vi "Sort 2D-Array.vi"(1 "Sort Order (0->9)":enum16{"0 --> 9", "9 --> 0"}(ring), 2 "Search Parameters":T1, 7 "2D-String-Array_in":string[][](array[string])=[["45245,25", "Hallo", "Eier"], ["45245,36", "Ballo", "Mehl"], ["45245,84", "Lallo", "Zucker"], ["245", "Trallo", "Salz"], ["45", "Knallo", "Bier"]]) -> (8 "2D-String-Array_SortedByColumn":string[][](array[string]))   [LabVIEW 2022 SP3, in "hse-misc.lvlib"]
doc: "Sorts a 2D string array by the column declared in <b>Search parameters</b> and by <b>Sort Order</b>.\n\n\n\n____\nHAMPEL SOFTWARE ENGINEERING v3.8.0 (2023-12-18 14:41)"
uses:
  hse-misc.lvlib
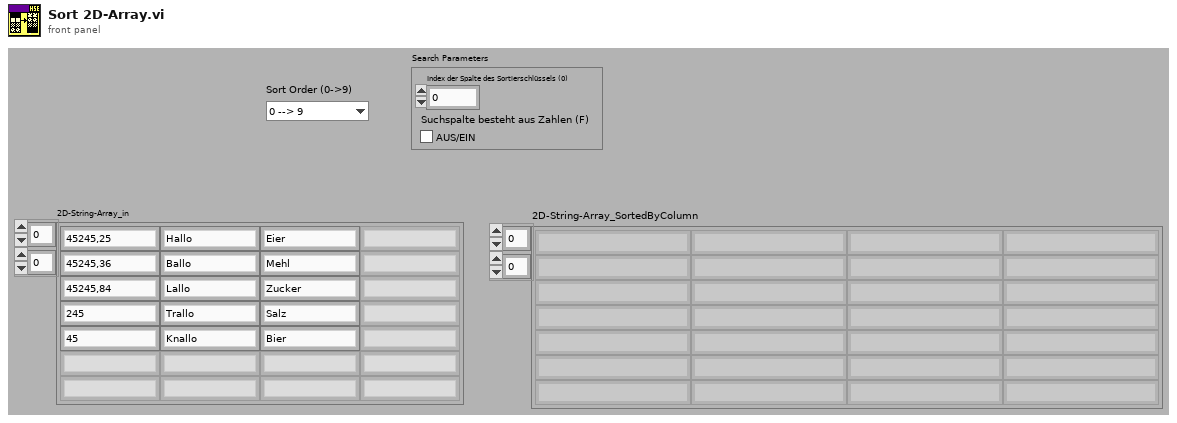
[diagram p1: front panel]
types:
  T1 = cluster{"Index der Spalte des Sortierschlüssels (0)":i32, "Suchspalte besteht aus Zahlen (F)":bool}
  T2 = cluster{"[0]":string, "[1]":string, "[2]":string, "[3]":string, "[4]":string, "[5]":string, "[6]":string, "[7]":string, "[8]":string, "[9]":string, "[10]":string, "[11]":string, "[12]":string, "[13]":string, "[14]":string, "[15]":string, "[16]":string, "[17]":string, "[18]":string, "[19]":string, "[20]":string, "[21]":string, "[22]":string, "[23]":string, "[24]":string, "[25]":string, "[26]":string, "[27]":string, "[28]":string, "[29]":string, "[30]":string, "[31]":string, "[32]":string, "[33]":string, "[34]":string, "[35]":string, "[36]":string, "[37]":string, "[38]":string, "[39]":string, "[40]":string, "[41]":string, "[42]":string, "[43]":string, "[44]":string, "[45]":string, "[46]":string, "[47]":string, "[48]":string, "[49]":string, "[50]":string, "[51]":string, "[52]":string, "[53]":string, "[54]":string, "[55]":string, "[56]":string, "[57]":string, "[58]":string, "[59]":string, "[60]":string, "[61]":string, "[62]":string, "[63]":string, "[64]":string, "[65]":string, "[66]":string, "[67]":string, "[68]":string, "[69]":string, "[70]":string, "[71]":string, "[72]":string, "[73]":string, "[74]":string, "[75]":string, "[76]":string, "[77]":string, "[78]":string, "[79]":string, "[80]":string, "[81]":string, "[82]":string, "[83]":string, "[84]":string, "[85]":string, "[86]":string, "[87]":string, "[88]":string, "[89]":string, "[90]":string, "[91]":string, "[92]":string, "[93]":string, "[94]":string, "[95]":string, "[96]":string, "[97]":string, "[98]":string, "[99]":string}
  T3 = cluster{dbl, cluster{"[0]":string, "[1]":string, "[2]":string, "[3]":string, "[4]":string, "[5]":string, "[6]":string, "[7]":string, "[8]":string, "[9]":string, "[10]":string, "[11]":string, "[12]":string, "[13]":string, "[14]":string, "[15]":string, "[16]":string, "[17]":string, "[18]":string, "[19]":string, "[20]":string, "[21]":string, "[22]":string, "[23]":string, "[24]":string, "[25]":string, "[26]":string, "[27]":string, "[28]":string, "[29]":string, "[30]":string, "[31]":string, "[32]":string, "[33]":string, "[34]":string, "[35]":string, "[36]":string, "[37]":string, "[38]":string, "[39]":string, "[40]":string, "[41]":string, "[42]":string, "[43]":string, "[44]":string, "[45]":string, "[46]":string, "[47]":string, "[48]":string, "[49]":string, "[50]":string, "[51]":string, "[52]":string, "[53]":string, "[54]":string, "[55]":string, "[56]":string, "[57]":string, "[58]":string, "[59]":string, "[60]":string, "[61]":string, "[62]":string, "[63]":string, "[64]":string, "[65]":string, "[66]":string, "[67]":string, "[68]":string, "[69]":string, "[70]":string, "[71]":string, "[72]":string, "[73]":string, "[74]":string, "[75]":string, "[76]":string, "[77]":string, "[78]":string, "[79]":string, "[80]":string, "[81]":string, "[82]":string, "[83]":string, "[84]":string, "[85]":string, "[86]":string, "[87]":string, "[88]":string, "[89]":string, "[90]":string, "[91]":string, "[92]":string, "[93]":string, "[94]":string, "[95]":string, "[96]":string, "[97]":string, "[98]":string, "[99]":string}}
  T4 = cluster{dbl, cluster{"[0]":string, "[1]":string, "[2]":string, "[3]":string, "[4]":string, "[5]":string, "[6]":string, "[7]":string, "[8]":string, "[9]":string, "[10]":string, "[11]":string, "[12]":string, "[13]":string, "[14]":string, "[15]":string, "[16]":string, "[17]":string, "[18]":string, "[19]":string, "[20]":string, "[21]":string, "[22]":string, "[23]":string, "[24]":string, "[25]":string, "[26]":string, "[27]":string, "[28]":string, "[29]":string, "[30]":string, "[31]":string, "[32]":string, "[33]":string, "[34]":string, "[35]":string, "[36]":string, "[37]":string, "[38]":string, "[39]":string, "[40]":string, "[41]":string, "[42]":string, "[43]":string, "[44]":string, "[45]":string, "[46]":string, "[47]":string, "[48]":string, "[49]":string, "[50]":string, "[51]":string, "[52]":string, "[53]":string, "[54]":string, "[55]":string, "[56]":string, "[57]":string, "[58]":string, "[59]":string, "[60]":string, "[61]":string, "[62]":string, "[63]":string, "[64]":string, "[65]":string, "[66]":string, "[67]":string, "[68]":string, "[69]":string, "[70]":string, "[71]":string, "[72]":string, "[73]":string, "[74]":string, "[75]":string, "[76]":string, "[77]":string, "[78]":string, "[79]":string, "[80]":string, "[81]":string, "[82]":string, "[83]":string, "[84]":string, "[85]":string, "[86]":string, "[87]":string, "[88]":string, "[89]":string, "[90]":string, "[91]":string, "[92]":string, "[93]":string, "[94]":string, "[95]":string, "[96]":string, "[97]":string, "[98]":string, "[99]":string}}[]
  T5 = cluster{"[0]":string, "[1]":string, "[2]":string, "[3]":string, "[4]":string, "[5]":string, "[6]":string, "[7]":string, "[8]":string, "[9]":string, "[10]":string, "[11]":string, "[12]":string, "[13]":string, "[14]":string, "[15]":string, "[16]":string, "[17]":string, "[18]":string, "[19]":string, "[20]":string, "[21]":string, "[22]":string, "[23]":string, "[24]":string, "[25]":string, "[26]":string, "[27]":string, "[28]":string, "[29]":string, "[30]":string, "[31]":string, "[32]":string, "[33]":string, "[34]":string, "[35]":string, "[36]":string, "[37]":string, "[38]":string, "[39]":string, "[40]":string, "[41]":string, "[42]":string, "[43]":string, "[44]":string, "[45]":string, "[46]":string, "[47]":string, "[48]":string, "[49]":string, "[50]":string, "[51]":string, "[52]":string, "[53]":string, "[54]":string, "[55]":string, "[56]":string, "[57]":string, "[58]":string, "[59]":string, "[60]":string, "[61]":string, "[62]":string, "[63]":string, "[64]":string, "[65]":string, "[66]":string, "[67]":string, "[68]":string, "[69]":string, "[70]":string, "[71]":string, "[72]":string, "[73]":string, "[74]":string, "[75]":string, "[76]":string, "[77]":string, "[78]":string, "[79]":string, "[80]":string, "[81]":string, "[82]":string, "[83]":string, "[84]":string, "[85]":string, "[86]":string, "[87]":string, "[88]":string, "[89]":string, "[90]":string, "[91]":string, "[92]":string, "[93]":string, "[94]":string, "[95]":string, "[96]":string, "[97]":string, "[98]":string, "[99]":string}[]
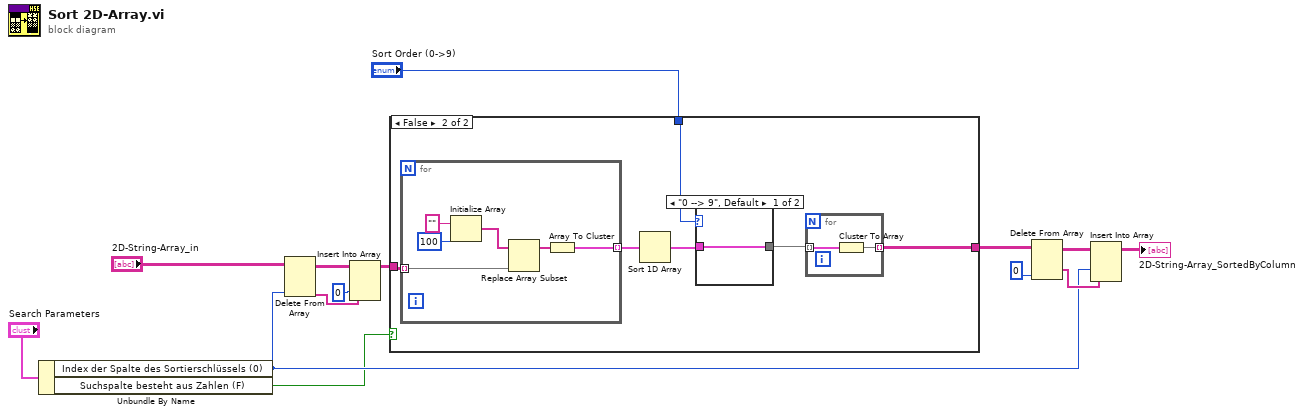
[diagram p0: block diagram]
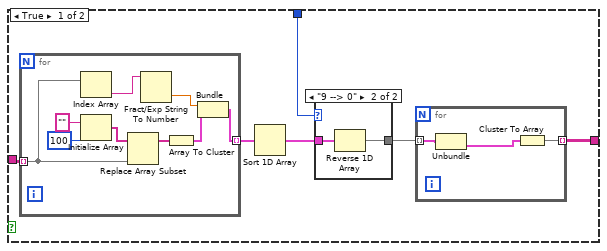
[diagram p2: hidden frame]
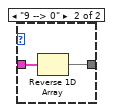
[diagram p4: hidden frame]
diagram:
  n1 = Unbundle By Name("Search Parameters") -> ("Index der Spalte des Sortierschlüssels (0)"=w4:i32, "Suchspalte besteht aus Zahlen (F)"=w3:bool)
  n2 = Delete From Array(array="2D-String-Array_in", index (col)=w4) -> (deleted portion=w6:string[], array with subset deleted=w14:string[][])  [unwired: 2 in]
  n3 = Insert Into Array(array=w14, index (col)=0 ("Deaktivierter Index (Spalte)"), new element=w6) -> (w12:string[][])  [unwired: 1 in]
  n4 = case shown="False" w3 {
    tunnel: w12 -> [w18 w40]
    tunnel: [w17 w39] -> w8
    tunnel: "Sort Order (0->9)" -> [w15 w36]
    frame True {
      n5 = for {
        tunnel: w18 -> [w28] mode=indexing
        tunnel: [w25] -> w20 mode=indexing
        n6 = Index Array(array=w28) -> (element=w27:string)  [unwired: 1 in]
        n7 = Initialize Array("", 100 ("Dimensionsgröße")) -> (w30:string[])
        n8 = Replace Array Subset(array=w30, new element=w28) -> (w29:string[])  [unwired: 1 in]
        n9 = Fract/Exp String To Number(string=w27) -> (number=w24:dbl)  [unwired: 3 in, 1 out]
        n10 = Array To Cluster(array=w29) -> (cluster=w26:T2)
        n11 = Bundle(w24, w26) -> (w25:T3)  [unwired: 1 in]
      }
      n12 = Sort 1D Array(array=w20) -> (sorted array=w19:T4)
      n13 = case shown="\"9 --> 0\"" w15 {
        tunnel: w19 -> [w21 w23]
        tunnel: [w21 w22] -> w16
        frame "0 --> 9", Default {
        }
        frame "9 --> 0" {
          n14 = Reverse 1D Array(array=w23) -> (reversed array=w22:T4)
        }
      }
      n15 = for {
        tunnel: w16 -> [w34] mode=indexing
        tunnel: [w35] -> w17 mode=indexing
        n16 = Unbundle(w34) -> (w33:T2)  [unwired: 1 out]
        n17 = Cluster To Array(cluster=w33) -> (array=w35:string[])
      }
    }
    frame False {
      n18 = for {
        tunnel: w40 -> [w46] mode=indexing
        tunnel: [w45] -> w41 mode=indexing
        n19 = Initialize Array("", 100 ("Dimensionsgröße")) -> (w48:string[])
        n20 = Replace Array Subset(array=w48, new element=w46) -> (w47:string[])  [unwired: 1 in]
        n21 = Array To Cluster(array=w47) -> (cluster=w45:T2)
      }
      n22 = Sort 1D Array(array=w41) -> (sorted array=w38:T5)
      n23 = case shown="\"0 --> 9\", Default" w36 {
        tunnel: w38 -> [w42 w44]
        tunnel: [w42 w43] -> w37
        frame "0 --> 9", Default {
        }
        frame "9 --> 0" {
          n24 = Reverse 1D Array(array=w44) -> (reversed array=w43:T5)
        }
      }
      n25 = for {
        tunnel: w37 -> [w52] mode=indexing
        tunnel: [w51] -> w39 mode=indexing
        n26 = Cluster To Array(cluster=w52) -> (array=w51:string[])
      }
    }
  }
  n27 = Delete From Array(array=w8, index (col)=0 ("Deaktivierter Index (Spalte)")) -> (deleted portion=w11:string[], array with subset deleted=w10:string[][])  [unwired: 2 in]
  n28 = Insert Into Array(array=w10, index (col)=w4, new element=w11) -> (→"2D-String-Array_SortedByColumn":string[][])  [unwired: 1 in]
